vi "execute.vi"(8 "error in (no error)":errorcluster, 9 "trajectory in":refnum<class "GenericComponent.lvclass">, 10 "imaging mode in":refnum<class "GenericComponent.lvclass">, 11 "DL090310ImagingModeToTrajectoryAdapter in":refnum<class "AdapterDL090310ImagingModeToTrajectory.lvclass">) -> (0 "error out":errorcluster, 1 "trajectory out":refnum<class "GenericComponent.lvclass">, 2 "imaging mode out":refnum<class "GenericComponent.lvclass">, 3 "DL090310ImagingModeToTrajectoryAdapter out":refnum<class "AdapterDL090310ImagingModeToTrajectory.lvclass">)   [LabVIEW 2010, in "AdapterDL090310ImagingModeToTrajectory.lvclass"]
uses:
  AdapterDL090310ImagingModeToTrajectory.lvclass
  common/classes/GenericComponent/GenericComponent/GenericComponent.lvclass
  Trajectory/TrajectoryDL090201FrameScan/TrajectoryDL090201FrameScan/speed_param_enum.ctl
  Trajectory/TrajectoryDL090201FrameScan/TrajectoryDL090201FrameScan/TrajectoryDL090201FrameScan.lvclass
  ImagingMode/ImagingModeDL090130Frame/ImagingModeDL090130Frame/ImagingModeDL090130Frame.lvclass
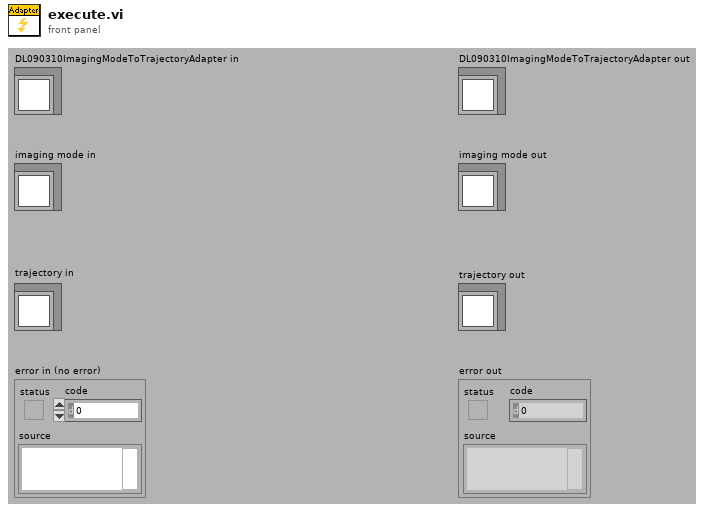
[diagram p1: front panel]
types:
  T1 = typedef "TrajectoryDL090201FrameScan.lvclass/speed_param_enum.ctl" = enum16{"frame rate", "line-scan time", "pixel-dwell time"}
  T2 = typedef "ImagingModeDL090130Frame.lvclass/speed_parameter_cluster.ctl" = enum16{"frame rate", "line-scan time", "pixel-dwell time"}
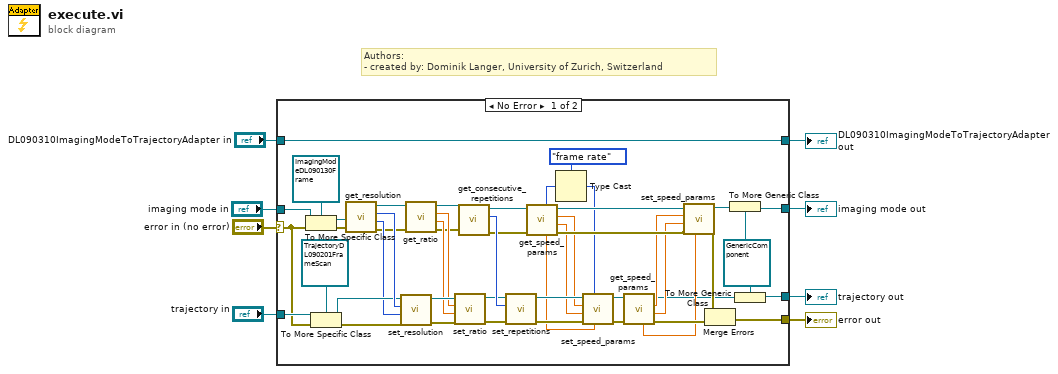
[diagram p0: block diagram]
diagram:
  # "Authors: \n- created by: Dominik Langer, University of Zurich, Switzerland"
  n1 = case shown="No Error" "error in (no error)" {
    selector: "error in (no error)" -> [w35 w60]
    tunnel: [w25 w60] -> w7
    tunnel: [w47 w59] -> w5
    tunnel: "DL090310ImagingModeToTrajectoryAdapter in" -> [w47 w59]
    tunnel: "imaging mode in" -> [w50 w58]
    tunnel: "trajectory in" -> [w49 w57]
    tunnel: [w48 w58] -> w2
    tunnel: [w46 w57] -> w1
    frame No Error {
      w13 = refnum<class "GenericComponent.lvclass"> refnum ("GenericComponent.lvclass")
      n2 = To More Specific Class(target class=refnum<class "ImagingModeDL090130Frame.lvclass"> refnum ("DL090130FrameScanMode.lvclass"), reference=w50, error in=w35) -> (specific class reference=w53:refnum<class "ImagingModeDL090130Frame.lvclass">, error out=w33:errorcluster)
      n3 = To More Specific Class(target class=refnum<class "TrajectoryDL090201FrameScan.lvclass"> refnum ("TrajectoryDL090201FrameScan.lvclass"), reference=w49, error in=w35) -> (specific class reference=w52:refnum<class "TrajectoryDL090201FrameScan.lvclass">, error out=w34:errorcluster)
      n4 = call-dynamic "get_resolution.vi"("error in (no error)"=w33, "ImagingModeDL090130Frame in"=w53) -> ("error out"=w32:errorcluster, "y resolution"=w45:i32, "x resolution"=w54:i32, "ImagingModeDL090130Frame out"=w40:refnum<class "ImagingModeDL090130Frame.lvclass">)  [unwired: 6 out]
      n5 = call-dynamic "set_resolution.vi"("error in (no error)"=w34, "y"=w45, "x"=w54, "TrajectoryDL090201FrameScan in"=w52) -> ("error out"=w31:errorcluster, "TrajectoryDL090201FrameScan out"=w44:refnum<class "TrajectoryDL090201FrameScan.lvclass">)  [unwired: 6 out]
      n6 = call-dynamic "get_ratio.vi"("error in (no error)"=w32, "ImagingModeDL090130Frame in"=w40) -> ("error out"=w30:errorcluster, "y ratio factor"=w41:dbl, "x ratio factor"=w42:dbl, "ImagingModeDL090130Frame out"=w39:refnum<class "ImagingModeDL090130Frame.lvclass">)  [unwired: 6 out]
      n7 = call-dynamic "set_ratio.vi"("error in (no error)"=w31, "y"=w41, "x"=w42, "TrajectoryDL090201FrameScan in"=w44) -> ("error out"=w29:errorcluster, "TrajectoryDL090201FrameScan out"=w43:refnum<class "TrajectoryDL090201FrameScan.lvclass">)  [unwired: 6 out]
      n8 = call-dynamic "get_consecutive_repetitions.vi"("error in (no error)"=w30, "ImagingModeDL090130Frame in"=w39) -> ("error out"=w28:errorcluster, "number of consecutive repetitions"=w51:i32, "ImagingModeDL090130Frame out"=w38:refnum<class "ImagingModeDL090130Frame.lvclass">)  [unwired: 7 out]
      n9 = call-dynamic "set_repetitions.vi"("error in (no error)"=w29, "repetitions"=w51, "GenericTrajectory in"=w43) -> ("error out"=w19:errorcluster, "GenericTrajectory out"=w16:refnum<class "TrajectoryDL090201FrameScan.lvclass">)  [unwired: 7 out]
      n10 = call-dynamic "get_speed_params.vi"("error in (no error)"=w28, "ImagingModeDL090130Frame in"=w38) -> ("error out"=w27:errorcluster, "line-scan time"=w14:dbl[unit], "frame rate"=w15:dbl[unit], "ImagingModeDL090130Frame out"=w36:refnum<class "ImagingModeDL090130Frame.lvclass">, "pixel dwell time"=w12:dbl[unit], "which one is correct for sure?"=w10:T2)  [unwired: 4 in]
      n11 = Type Cast(type=speed_param_enum."frame rate" ("speed param"), x=w10) -> (*(type *) &x=w9:T1)
      n12 = call-dynamic "set_speed_params.vi"("pixel-dwell time"=w12, "speed param"=w9, "error in (no error)"=w19, "line-scan time"=w14, "frame rate"=w15, "TrajectoryDL090201FrameScan in"=w16) -> ("error out"=w18:errorcluster, "TrajectoryDL090201FrameScan out"=w17:refnum<class "TrajectoryDL090201FrameScan.lvclass">)  [unwired: 4 in]
      n13 = call-dynamic "get_speed_params.vi"("error in (no error)"=w18, "TrajectoryDL090201FrameScan in"=w17) -> ("error out"=w24:errorcluster, "line-scan time"=w22:dbl[unit], "frame rate"=w23:dbl[unit], "TrajectoryDL090201FrameScan out"=w20:refnum<class "TrajectoryDL090201FrameScan.lvclass">, "pixel-dwell time"=w21:dbl[unit])  [unwired: 5 in]
      n14 = call-dynamic "set_speed_params.vi"("pixel-dwell time"=w21, "error in (no error)"=w27, "line-scan time"=w22, "frame rate"=w23, "ImagingModeDL090130Frame in"=w36) -> ("error out"=w26:errorcluster, "ImagingModeDL090130Frame out"=w37:refnum<class "ImagingModeDL090130Frame.lvclass">)  [unwired: 5 in]
      n15 = Merge Errors(w26, w24) -> (w25:errorcluster)
      n16 = To More Generic Class(target class=w13, reference=w37) -> (generic class reference=w48:refnum<class "GenericComponent.lvclass">)
      n17 = To More Generic Class(target class=w13, reference=w20) -> (generic class reference=w46:refnum<class "GenericComponent.lvclass">)
    }
    frame Error {
    }
  }
  "error out" <- w7
  "DL090310ImagingModeToTrajectoryAdapter out" <- w5
  "imaging mode out" <- w2
  "trajectory out" <- w1
